vi "FarfieldGeneratePosgrid.vi"() -> (0 "error out":errorcluster caption="错误输出", 2 "posOut":cluster{"俯仰":dbl, "旋转":dbl}[][](array[cluster]), 3 "Reference Grid":cluster{"数组":i32[], "数组":i32[]})   [LabVIEW 2018]
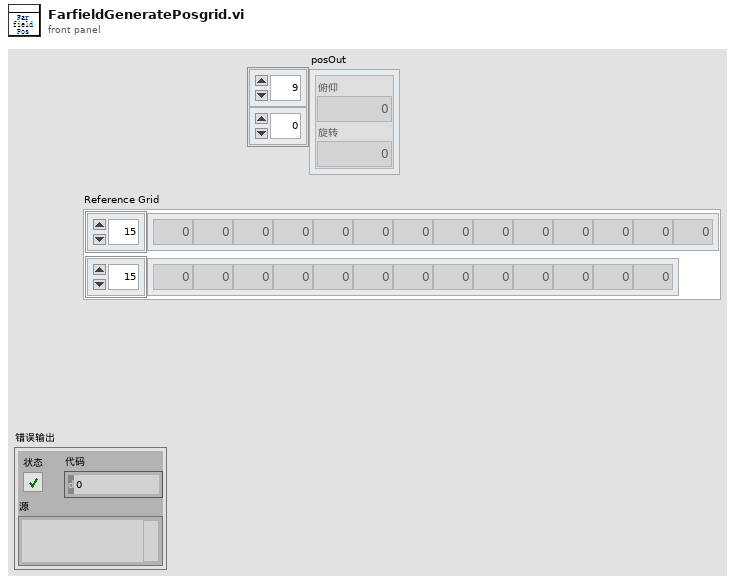
[diagram p1: front panel]
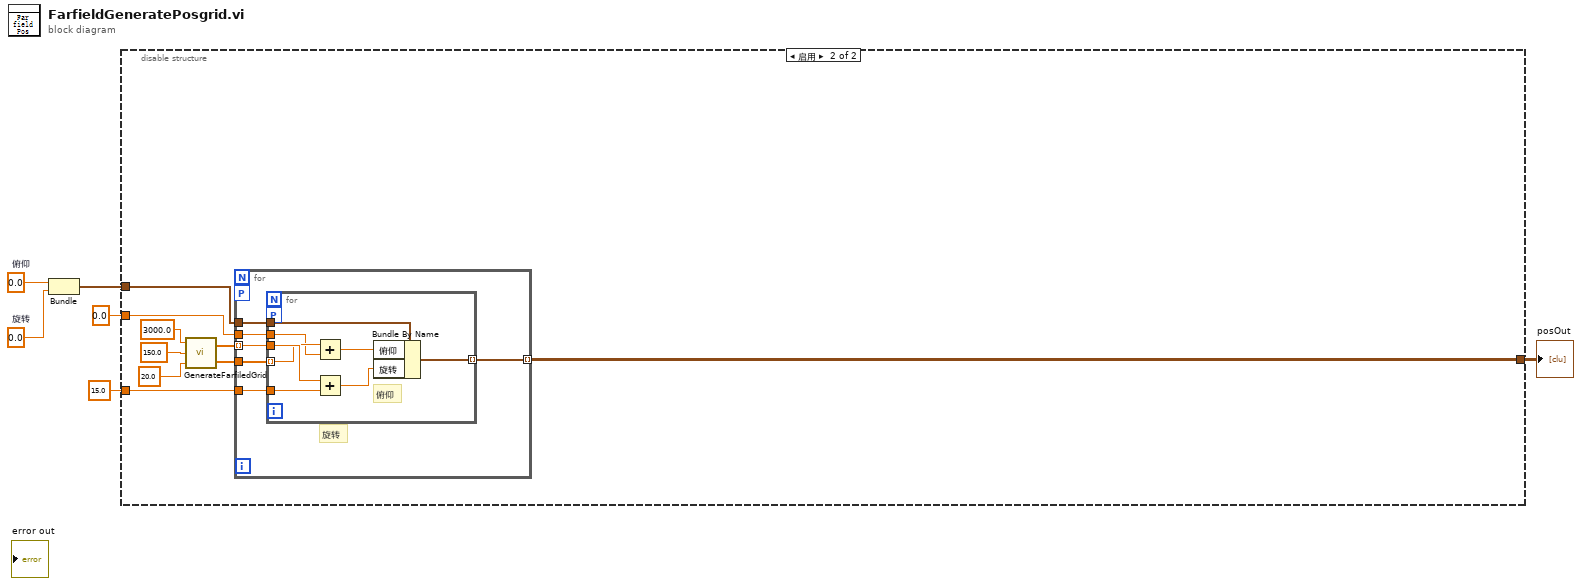
[diagram p0: block diagram]
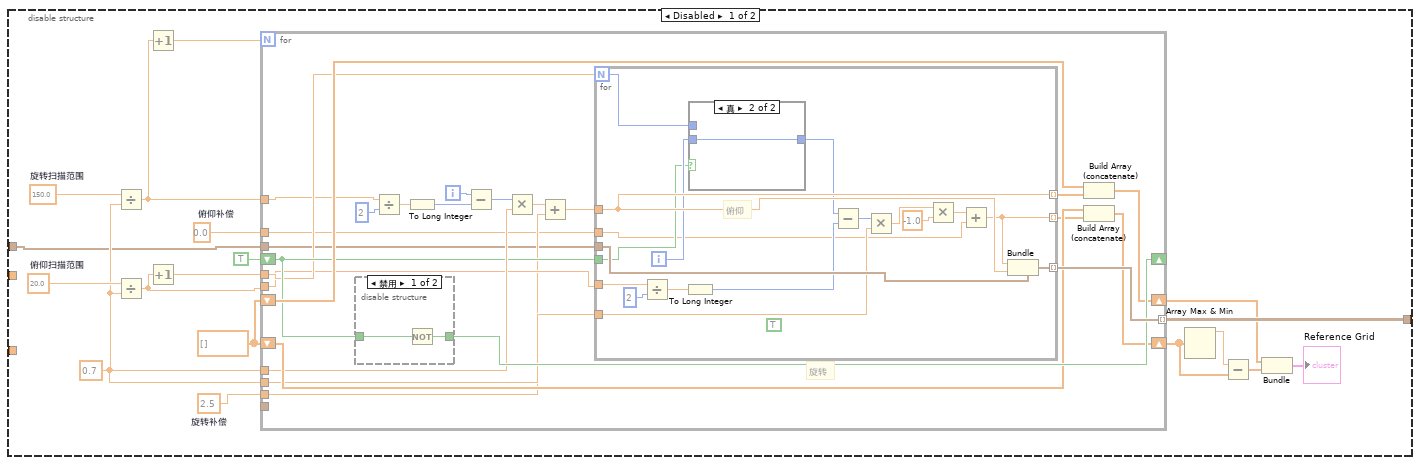
[diagram p2: hidden frame]
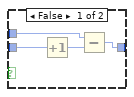
[diagram p4: hidden frame]
diagram:
  w3 = 0.0  # 旋转
  w4 = 0.0  # 俯仰
  n1 = Bundle("俯仰"=w4, "旋转"=w3) -> (w5:cluster{"俯仰":dbl, "旋转":dbl})  [unwired: 1 in]
  n2 = disable-structure shown="启用" {
    disable-tunnel: [w24 w78] -> w6
    disable-tunnel: w5 -> [w7 w79]
    disable-tunnel: 15.0 -> [_ w77]
    disable-tunnel: 0.0 -> [_ w76]
    frame Disabled {
      w8 = 0.0  # 俯仰补偿
      w9 = 2.5  # 旋转补偿
      w14 = 0.7
      w15 = 20.0  # 俯仰扫描范围
      w16 = 150.0  # 旋转扫描范围
      w22 = dbl[] []
      n3 = Divide(x=w16, y=w14) -> (x/y=w11:dbl)
      n4 = Divide(x=w15, y=w14) -> (x/y=w10:dbl)
      n5 = Increment(x=w11) -> (x+1=w13:dbl)
      n6 = Increment(x=w10) -> (x+1=w12:dbl)
      n7 = for {
        N: w13 -> [_]
        tunnel: [w49] -> w24 mode=indexing
        shift-right: [w48] -> _
        shift-left: TRUE -> [w36]
        shift-right: [w45] -> w20
        shift-left: w22 -> [w46]
        shift-right: [w43] -> w18
        shift-left: w22 -> [w44]
        tunnel: _ -> [w42]
        tunnel: w14 -> [w40]
        tunnel: w14 -> [w39]
        tunnel: w12 -> [w32]
        tunnel: w11 -> [w31]
        tunnel: w10 -> [w30]
        tunnel: w9 -> [w27]
        tunnel: w8 -> [w26]
        tunnel: w7 -> [w25]
        i -> [w35]
        # "旋转"
        n8 = disable-structure shown="禁用" {
          disable-tunnel: [w51 w52] -> w48
          disable-tunnel: w36 -> [w50 w52]
          frame Disabled {
            n9 = Not(x=w50) -> (.not. x?=w51:bool)
          }
          frame Enabled {
          }
        }
        n10 = Divide(x=w31, y=2) -> (x/y=w37:dbl)
        n11 = To Long Integer(number=w37) -> (32bit integer=w33:i32)
        n12 = Subtract(x=w35, y=w33) -> (x-y=w41:i32)
        n13 = Multiply(x=w41, y=w40) -> (x*y=w28:dbl)
        n14 = Add(x=w28, y=w27) -> (x+y=w29:dbl)
        n15 = for {
          N: w32 -> [w62]
          tunnel: w29 -> [w69]
          tunnel: [w70] -> w49 mode=indexing
          tunnel: [w69] -> w47 mode=indexing
          tunnel: [w55] -> w34 mode=indexing
          tunnel: w25 -> [w68]
          tunnel: w39 -> [w66]
          tunnel: w36 -> [w56]
          tunnel: w30 -> [w58]
          tunnel: w26 -> [w53]
          i -> [w63]
          (unwired) TRUE
          # "俯仰"
          n16 = Divide(x=w58, y=2) -> (x/y=w64:dbl)
          n17 = To Long Integer(number=w64) -> (32bit integer=w59:i32)
          n18 = case shown="真" w56 {
            tunnel: w63 -> [w74 w75]
            tunnel: w62 -> [w73 _]
            tunnel: [w71 w75] -> w61
            frame False {
              n19 = Increment(x=w74) -> (x+1=w72:i32)
              n20 = Subtract(x=w73, y=w72) -> (x-y=w71:i32)
            }
            frame True {
            }
          }
          n21 = Subtract(x=w61, y=w59) -> (x-y=w67:i32)
          n22 = Multiply(x=w67, y=w66) -> (x*y=w60:dbl)
          n23 = Multiply(x=w60, y=-1.0) -> (x*y=w54:dbl)
          n24 = Add(x=w54, y=w53) -> (x+y=w55:dbl)
          n25 = Bundle(cluster=w68, "俯仰"=w55, "旋转"=w69) -> (w70:cluster{"俯仰":dbl, "旋转":dbl})
        }
        n26 = Build Array (concatenate)(w46, w47) -> (w45:dbl[])
        n27 = Build Array (concatenate)(w44, w34) -> (w43:dbl[])
      }
      n28 = Array Max & Min(array=w18) -> (max value=w19:dbl)  [unwired: 3 out]
      n29 = Subtract(x=w19, y=w18) -> (x-y=w17:dbl[])
      n30 = Bundle(w20, w17) -> (→"Reference Grid":cluster{dbl[], dbl[]})  [unwired: 1 in]
    }
    frame Enabled {
      n31 = call "GenerateFarfiledGrid.vi"("thetaPicth"=20.0, "thetaRol"=150.0, "L"=3000.0) -> ("PitchGrid"=w80:dbl[], "RollGrid"=w81:dbl[])  [unwired: 1 in]
      n32 = for "For循环" {
        tunnel: w81 -> [w88] mode=indexing
        tunnel: w80 -> [w90]
        tunnel: w79 -> [w89]
        tunnel: [w87] -> w78 mode=indexing
        tunnel: w77 -> [w86]
        tunnel: w76 -> [w85]
        workers-P: _ -> [_]
        # "旋转"
        n33 = for "For循环" {
          tunnel: w90 -> [w93] mode=indexing
          tunnel: w89 -> [w98]
          tunnel: w88 -> [w95]
          tunnel: [w97] -> w87 mode=indexing
          tunnel: w86 -> [w94]
          tunnel: w85 -> [w92]
          workers-P: _ -> [_]
          # "俯仰"
          n34 = Add(x=w93, y=w92) -> (x+y=w91:dbl)
          n35 = Add(x=w95, y=w94) -> (x+y=w96:dbl)
          n36 = Bundle By Name(cluster=w98, "俯仰"=w91, "旋转"=w96) -> (w97:cluster{"俯仰":dbl, "旋转":dbl})
        }
      }
    }
  }
  "posOut" <- w6
